vi "testDemo2.vi"(8 "error in (no error)":errorcluster, 11 "MyFirstTest.lvclass in":refnum<class "LocationOutsideClassRoot.lvclass">) -> (0 "error out":errorcluster, 3 "MyFirstTest.lvclass out":refnum<class "LocationOutsideClassRoot.lvclass">)   [LabVIEW 2011, in "LocationOutsideClassRoot.lvclass"]
doc: "This VI is a demo test -- it ensures that \"dog\" != \"cat\""
uses:
  LocationOutsideClassRoot.lvclass
panel:
  # "Copyright © 2007 James Kring, Inc. All rights reserved.\n\nAuthor: Jim Kring [jim.kring@jameskring.com]\n\nThis library is provided \"AS IS\" ,WITHOUT WARRANTIES OR \nCONDITIONS OF ANY KIND, either express or implied.\n\nJames Kring, Inc. -- http://www.jameskring.com"
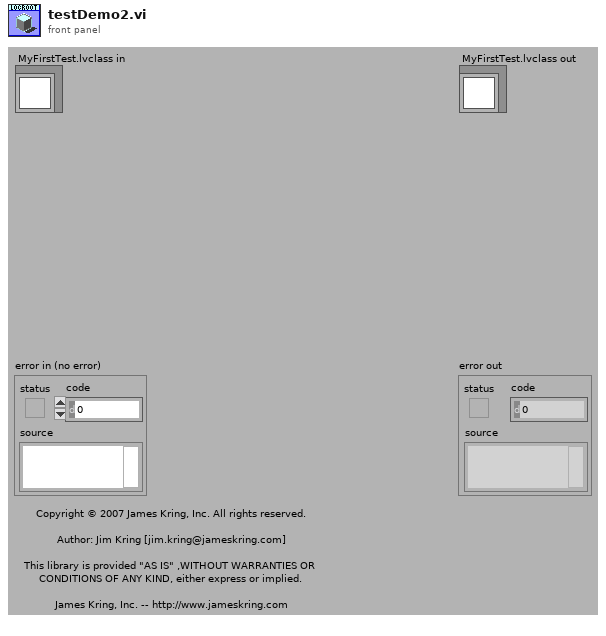
[diagram p1: front panel]
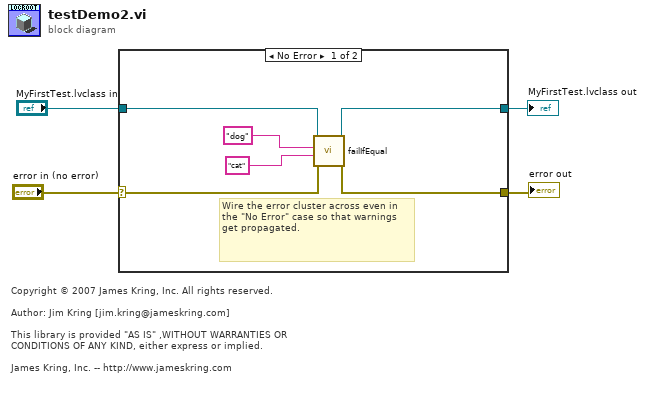
[diagram p0: block diagram]
diagram:
  # "Copyright © 2007 James Kring, Inc. All rights reserved.\n\nAuthor: Jim Kring [jim.kring@jameskring.com]\n\nThis library is provided \"AS IS\" ,WITHOUT WARRANTIES OR \nCONDITIONS OF ANY KIND, either express or implied.\n\nJames Kring, Inc. -- http://www.jameskring.com"
  n1 = case shown="No Error" "error in (no error)" {
    selector: "error in (no error)" -> [w6 w12]
    tunnel: [w5 w12] -> w3
    tunnel: [w7 w11] -> w1
    tunnel: "MyFirstTest.lvclass in" -> [w8 w11]
    frame No Error {
      # "Wire the error cluster across even in the \"No Error\" case so that warnings get propagated."
      n2 = call-dynamic "failIfEqual.vi"("error in (no error)"=w6, "y"="cat", "x"="dog", "TestCase in"=w8) -> ("error out"=w5:errorcluster, "TestCase out"=w7:refnum<class "LocationOutsideClassRoot.lvclass">)  [unwired: 6 in]
    }
    frame Error {
    }
  }
  "error out" <- w3
  "MyFirstTest.lvclass out" <- w1
